vi "Get Item Property (Variant).vi"(8 "error in (no error)":errorcluster, 9 "Default Value":variant, 10 "Property Name":string, 11 "Item Ref in":T1 format="%.0x") -> (0 "error out":errorcluster, 1 "Value":variant, 3 "Item Ref out":T1 format="%.0x", 4 "Found?":bool)   [LabVIEW 2019, in "Custom Device API.lvlib"]
doc: "Returns the <B>Value</B> of a specific item <B>Property Name</B>. Properties do not inherit within a custom device, so <B>Item Ref in</B> must reference the specific item on which the property is set. \n\nFor instances with a <B>Default Value</B> input, the <B>Value</B> output returns this value if the <B>Property Name</B> is not found for the specified item. Wire data to the <B>Default Value</B> input to determine the polymorphic instance to use or manually select the instance."
uses:
  Custom Device API.lvlib
  Custom Device Item Ref.ctl
  Custom Device Offline Path.vi
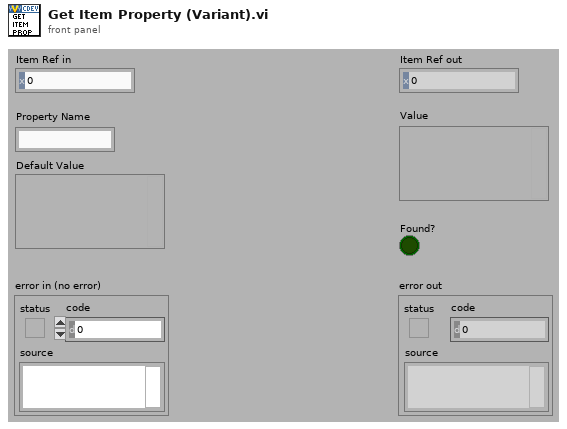
[diagram p1: front panel]
types:
  T1 = typedef "Custom Device API.lvlib/Custom Device Item Ref.ctl" = u64
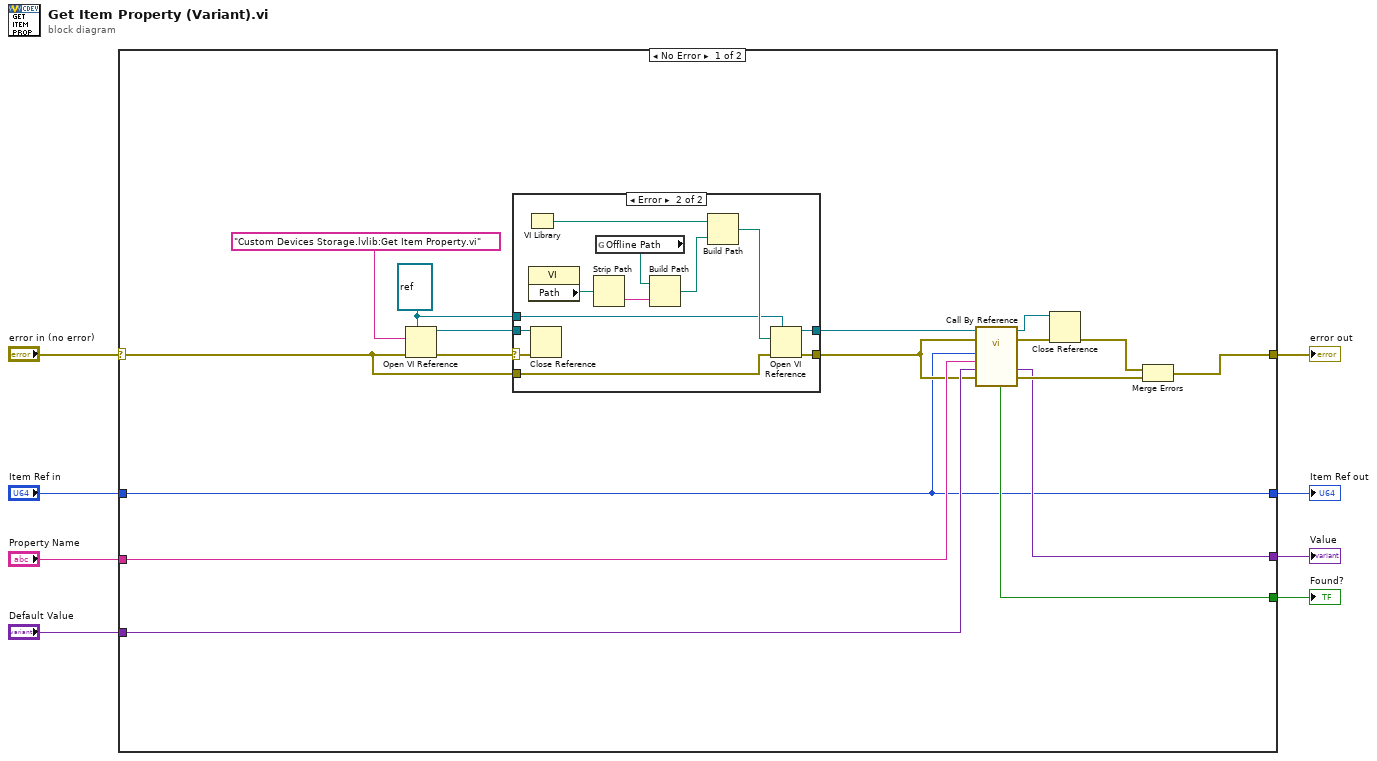
[diagram p0: block diagram]
diagram:
  n1 = case shown="No Error" "error in (no error)" {
    selector: "error in (no error)" -> [w18 w41]
    tunnel: [w24 w41] -> w8
    tunnel: "Item Ref in" -> [w17 w40]
    tunnel: "Property Name" -> [w23 _]
    tunnel: "Default Value" -> [w22 _]
    tunnel: [w17 w40] -> w4
    tunnel: [w21 _] -> w3
    tunnel: [w20 _] -> w2
    frame No Error {
      w11 = refnum<vi> refnum ("type specifier VI Refnum (for type only)")
      n2 = Open VI Reference(type specifier VI Refnum (for type only)=w11, vi path="Custom Devices Storage.lvlib:Get Item Property.vi", error in (no error)=w18) -> (vi reference=w12:refnum<vi>, error out=w13:errorcluster)  [unwired: 3 out]
      n3 = case shown="Error" w13 {
        selector: w13 -> [w27 w37]
        tunnel: w11 -> [_ w30]
        tunnel: w12 -> [w26 w38]
        tunnel: [w26 w36] -> w15
        tunnel: [w27 w35] -> w19
        tunnel: w18 -> [_ w39]
        frame No Error {
        }
        frame Error {
          n4 = VI Library() -> (path=w34:path)
          n5 = property class="VI"() -> ("Path"=w29:path)  [unwired: 2 in, 2 out]
          n6 = Close Reference(reference=w38, error in (no error)=w37) -> ()  [unwired: 1 out]
          n7 = Strip Path(path=w29) -> (name=w28:string)  [unwired: 1 out]
          n8 = global read "Custom Device Offline Path.vi" "Offline Path"() -> (w31:path)
          n9 = Build Path(base path=w31, name or relative path=w28) -> (appended path=w33:path)
          n10 = Build Path(base path=w34, name or relative path=w33) -> (appended path=w32:path)
          n11 = Open VI Reference(type specifier VI Refnum (for type only)=w30, vi path=w32, error in (no error)=w39) -> (vi reference=w36:refnum<vi>, error out=w35:errorcluster)  [unwired: 3 out]
        }
      }
      n12 = call-by-ref "?"(reference=w15, error in=w19, 8:"error in (no error)"=w19, "Default Value"=w22, "Property Name"=w23, "Item Ref in"=w17) -> (reference out=w9:refnum<vi>, error out=w16:errorcluster, 0:"error out"=w25:errorcluster, "Value"=w21:variant, "Found?"=w20:bool)  [unwired: 4 in, 1 out]
      n13 = Close Reference(reference=w9, error in (no error)=w16) -> (error out=w10:errorcluster)
      n14 = Merge Errors(w10, w25) -> (w24:errorcluster)
    }
    frame Error {
    }
  }
  "Item Ref out" <- w4
  "error out" <- w8
  "Value" <- w3
  "Found?" <- w2
